vi "Init Hardware.vi"(8 "error in (no error)":errorcluster, 11 "Instrument Driver in":refnum<class "Instrument Driver.lvclass">) -> (0 "error out":errorcluster, 3 "Instrument Driver out":refnum<class "Instrument Driver.lvclass">)   [LabVIEW 2015, in "Instrument Driver.lvclass"]
uses:
  Instrument Driver.lvclass
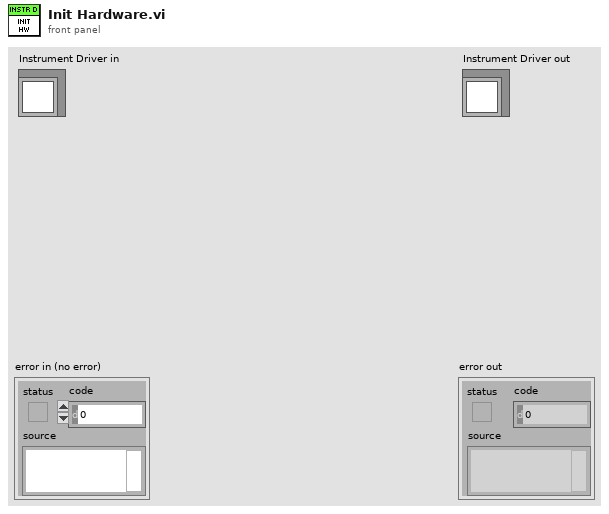
[diagram p1: front panel]
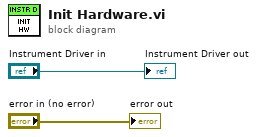
[diagram p0: block diagram]
diagram:
  "error out" <- "error in (no error)"
  "Instrument Driver out" <- "Instrument Driver in"
